vi "Evaluate Car Position Change.vi"(11 "Car Wash Station Sequencer in":refnum<class "Car Wash Station Sequencer.lvclass">) -> (3 "Car Wash Station Sequencer out":refnum<class "Car Wash Station Sequencer.lvclass">)   [LabVIEW 2016, in "CLD Exam - Car Wash.lvlib" / "Car Wash Station Sequencer.lvclass"]
uses:
  Car Wash Station Sequencer.lvclass
  D:/Repos/Stream/software/Mediator/Classes/Mediated Actor/Mediated Actor.lvclass
  Car Wash Station Sequencer.lvclass/Car Wash Station Sequencer.ctl
  Mediator/Classes/Message Interface/Message Interface.lvclass
  Mediator/Classes/Message Transport Queue/Message Transport Queue.lvclass
  Mediator/Classes/Mediated Actor/Mediated Actor.lvclass
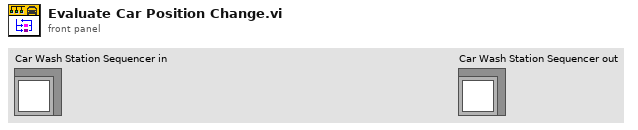
[diagram p1: front panel]
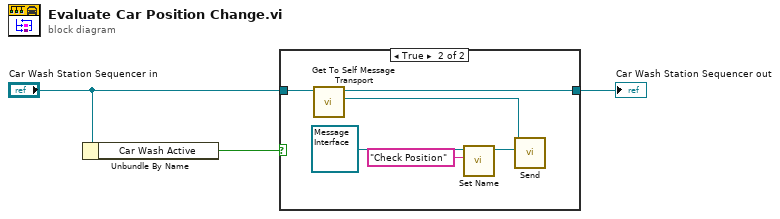
[diagram p0: block diagram]
diagram:
  n1 = Unbundle By Name("Car Wash Station Sequencer in") -> ("Car Wash Active"=w1:bool)
  n2 = case shown="True" w1 {
    tunnel: "Car Wash Station Sequencer in" -> [w4 w10]
    tunnel: [w4 w9] -> w2
    frame False {
    }
    frame True {
      n3 = call "Get To Self Message Transport.vi"("Mediated Actor in"=w10) -> ("To Self"=w8:refnum<class "Message Transport Queue.lvclass">, "Mediated Actor out"=w9:refnum<class "Car Wash Station Sequencer.lvclass">)  [unwired: 9 in]
      n4 = call "Set Name.vi"("Name"="Check Position", "Message Interface in"=refnum<class "Message Interface.lvclass"> refnum) -> ("Message Interface out"=w7:refnum<class "Message Interface.lvclass">)  [unwired: 8 in, 1 out]
      n5 = call-dynamic "Send.vi"("Message"=w7, "Message Transport Queue in"=w8) -> ()  [unwired: 7 in, 3 out]
    }
  }
  "Car Wash Station Sequencer out" <- w2
